vi "Omega_Read_Temp.vi"(8 "error in (no error)":errorcluster, 11 "VISA Omega (Serial - COM4)":refnum<visa-resource-name>) -> (0 "error out":errorcluster, 3 "value":dbl)   [LabVIEW 2012]
uses:
  <vilib>/Instr/_visa.llb/VISA Configure Serial Port (Instr).vi
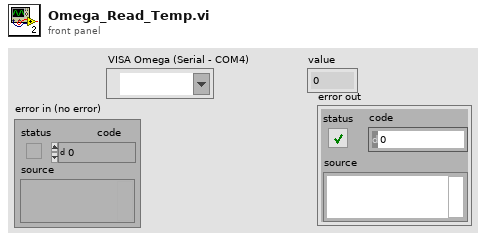
[diagram p1: front panel]
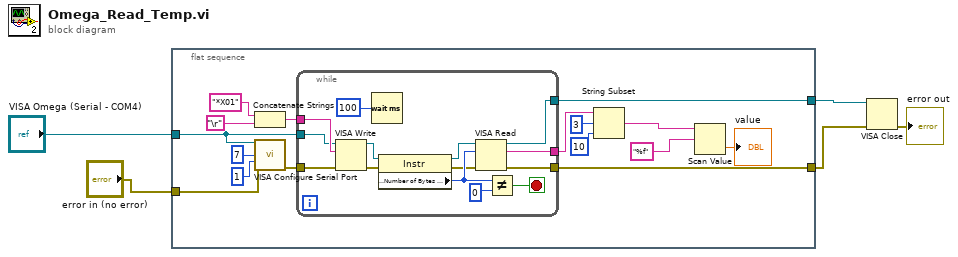
[diagram p0: block diagram]
diagram:
  n1 = flat-sequence {
    tunnel: "VISA Omega (Serial - COM4)" -> [w13]
    tunnel: [w11] -> w3
    tunnel: [w10] -> w4
    tunnel: "error in (no error)" -> [w6]
    frame #0 {
      n2 = Concatenate Strings("*X01", "\r") -> (w20:string)
      n3 = call-poly "VISA Configure Serial Port"("VISA resource name"=w13, "data bits (8)"=7, "parity (0:none)"=1, "error in (no error)"=w6) -> ("error out"=w17:errorcluster)  [unwired: 10 in, 1 out]
      n4 = while {
        tunnel: w20 -> [w35]
        tunnel: w17 -> [w34]
        tunnel: w13 -> [w33]
        tunnel: [w32] -> w12
        tunnel: [w31] -> w11
        tunnel: [w22] -> w10
        stop <- w24 stop-if-true
        n5 = VISA Write(VISA resource name=w33, write buffer=w35, error in (no error)=w34) -> (VISA resource name out=w30:refnum<visa-resource-name>, error out=w29:errorcluster)  [unwired: 1 out]
        n6 = Wait (ms)(milliseconds to wait=u32 100) -> ()  [unwired: 1 out]
        n7 = property class="Instr"(reference=w30, error in=w29) -> (reference out=w26:refnum<visa-resource-name>, error out=w25:errorcluster, "Serial Settings:Number of Bytes at Serial Port"=w27:u32)
        n8 = VISA Read(VISA resource name=w26, byte count=w27, error in (no error)=w25) -> (VISA resource name out=w22:refnum<visa-resource-name>, read buffer=w32:string, error out=w31:errorcluster)  [unwired: 1 out]
        n9 = Not Equal?(x=w27, y=u32 0) -> (x != y?=w24:bool)
      }
      n10 = String Subset(string=w12, offset (0)=3, length (rest)=10) -> (substring=w9:string)
      n11 = Scan Value(string=w9, format string="%f") -> (value=→"value":dbl)  [unwired: 1 in, 1 out]
    }
  }
  n12 = VISA Close(VISA resource name=w4, error in (no error)=w3) -> (error out=→"error out":errorcluster)
